vi "subSave_AcquireStageInfomation.vi"(3 "Positions":dbl[](array[numeric])=[55.78, 33.02, 0.0]) -> (1 "Text out":string)   [LabVIEW 2015]
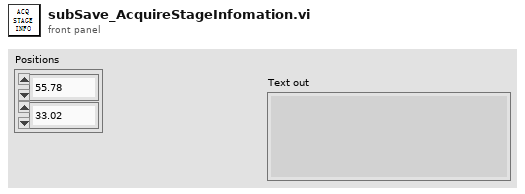
[diagram p1: front panel]
types:
  T1 = cluster{"Positions[0]":dbl, "Positions[1]":dbl, "Positions[2]":dbl, "Positions[3]":dbl, "Positions[4]":dbl, "Positions[5]":dbl, "Positions[6]":dbl, "Positions[7]":dbl, "Positions[8]":dbl}
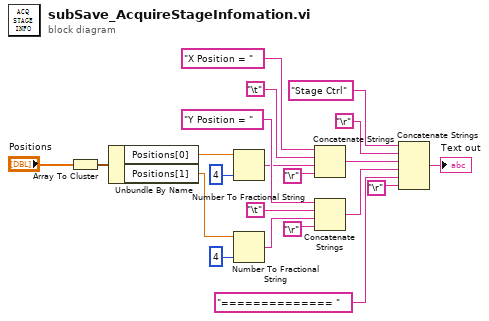
[diagram p0: block diagram]
diagram:
  n1 = Array To Cluster(array="Positions") -> (cluster=w3:T1)
  n2 = Unbundle By Name(w3) -> ("Positions[0]"=w6:dbl, "Positions[1]"=w7:dbl)
  n3 = Number To Fractional String(number=w6, precision (6)=i16 4) -> (F-format string=w10:string)  [unwired: 2 in]
  n4 = Number To Fractional String(number=w7, precision (6)=i16 4) -> (F-format string=w15:string)  [unwired: 2 in]
  n5 = Concatenate Strings("X Position = " ("string"), "\t", w10, "\r") -> (w18:string)
  n6 = Concatenate Strings("Y Position = " ("string"), "\t", w15, "\r") -> (w19:string)
  n7 = Concatenate Strings("Stage Ctrl" ("concatenated string"), "\r", w18, w19, "============== " ("string"), "\r") -> (→"Text out":string)
